vi "fp_window_properties.vi"() -> ()   [LabVIEW 2021]
uses:
  <vilib>/Utility/miscctls.llb/LVRectTypeDef.ctl
panel:
  out "Thermometer":dbl(slide)=45.91836734693878 scale=0.0..100.0
  out "2D Picture":picture
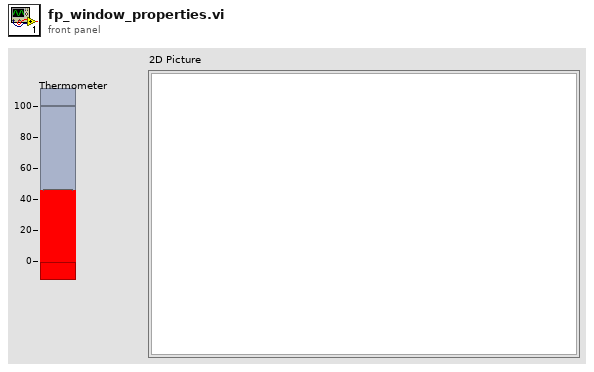
[diagram p1: front panel]
types:
  T1 = typedef "LVRectTypeDef.ctl" = cluster{"Left":i16, "Top":i16, "Right":i16, "Bottom":i16}
  T2 = typedef "imagedata.ctl" = cluster{"image type":i32, "image depth":i32, "image":u8[], "mask":u8[], "colors":u32[], "Rectangle":cluster{"left":i16, "top":i16, "right":i16, "bottom":i16}}
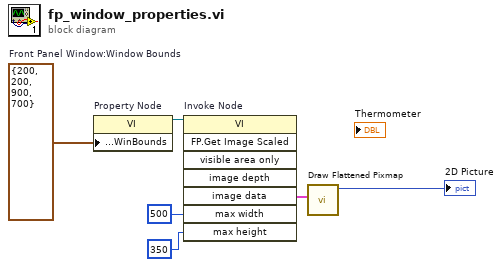
[diagram p0: block diagram]
diagram:
  w5 = T1 {"Left"=200, "Top"=200, "Right"=900, "Bottom"=700}  # Front Panel Window:Window Bounds
  n1 = property on="Property Node" class="VI"("Front Panel.WinBounds"=w5) -> (reference out=w2:refnum<vi>)  [unwired: 2 in, 1 out]
  n2 = invoke on="Invoke Node" class="VI" method="FP.Get Image Scaled"(reference=w2, "max width"=500 ("Maximum Width"), "max height"=350 ("Maximum Height")) -> ("image data"=w1:T2)  [unwired: 5 in, 7 out]
  n3 = call <vilib>:"Draw Flattened Pixmap.vi"("image data"=w1) -> ("new picture"=→"2D Picture":picture)  [unwired: 8 in]
